vi "GetDaysList.vi"(10 "month":string, 11 "year":string) -> (3 "Array":string[](array[string]))   [LabVIEW 2017, in "UI_TimeSelector.xctl"]
uses:
  UI_TimeSelector/UI_TimeSelector.xctl
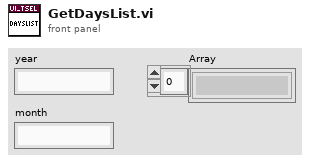
[diagram p1: front panel]
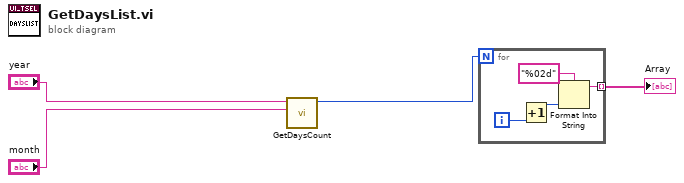
[diagram p0: block diagram]
diagram:
  n1 = call "GetDaysCount.vi"("month"="month", "year"="year") -> ("Numeric"=w3:i32)  [unwired: 9 in]
  n2 = for {
    N: w3 -> [_]
    tunnel: [w6] -> w1 mode=indexing
    i -> [w8]
    n3 = Increment(x=w8) -> (x+1=w7:i32)
    n4 = Format Into String(format string="%02d", w7) -> (resulting string=w6:string)  [unwired: 2 in, 1 out]
  }
  "Array" <- w1
